vi "Read Common Parameters from string.vi"(11 "String":string) -> (0 "error in (no error)":errorcluster, 3 "Script Parameters (common only)":map{string, string}(c390))   [LabVIEW 2020, in "Run Utilities.lvlib" / "Optimiser Cell.lvclass"]
uses:
  Optimiser Cell.lvclass
  Optimiser Cell.lvclass/Optimiser Cell.ctl
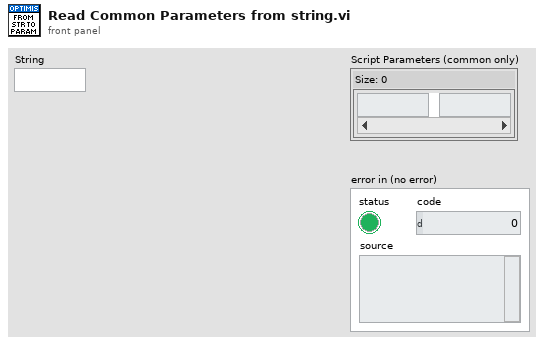
[diagram p1: front panel]
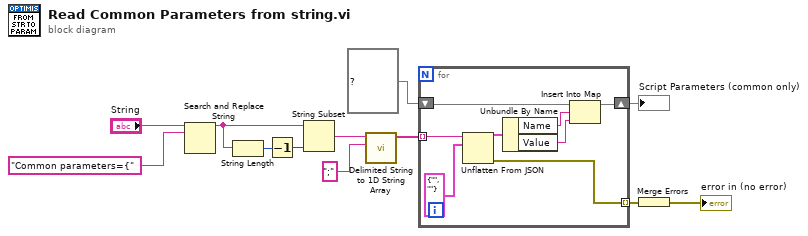
[diagram p0: block diagram]
diagram:
  n1 = Search and Replace String(input string="String", search string="Common parameters={" ("string")) -> (result string=w11:string)  [unwired: 6 in, 3 out]
  n2 = String Length(string=w11) -> (length=w10:i32)
  n3 = Decrement(x=w10) -> (x-1=w9:i32)
  n4 = String Subset(string=w11, length (rest)=w9) -> (substring=w8:string)  [unwired: 1 in]
  n5 = call <vilib>:"Delimited String to 1D String Array.vi"("delimiter"=";", "delimited string"=w8) -> ("string array"=w6:string[])  [unwired: 9 in]
  n6 = for {
    tunnel: [w20] -> w5 mode=indexing
    tunnel: w6 -> [w19] mode=indexing
    shift-right: [w17] -> w1
    shift-left: map{string, string} {} ("Script Parameters") -> [w16]
    n7 = Unflatten From JSON(JSON string=w19, type and defaults=cluster{"Name":string, "Value":string} {"Name"="", "Value"=""}) -> (value=w15:cluster{"Name":string, "Value":string}, error out=w20:errorcluster)  [unwired: 5 in]
    n8 = Unbundle By Name(w15) -> ("Name"=w14:string, "Value"=w13:string)
    n9 = Insert Into Map(map in=w16, key=w14, value=w13) -> (map out=w17:map{string, string})  [unwired: 2 out]
  }
  "Script Parameters (common only)" <- w1
  n10 = Merge Errors(w5) -> (→"error in (no error)":errorcluster)
